vi "WPI_DigitalOutputDisablePWM.vi"(8 "error in (no error)":errorcluster, 11 "DigitalOutputDevRef":T1={"DIO Channel"=enum."DIO 1", "DevStatus"={"status"=FALSE, "code"=0, "source"=""}}) -> (0 "error out":errorcluster, 3 "DigitalOutputDevRef":T1={"DIO Channel"=enum."DIO 1", "DevStatus"={"status"=FALSE, "code"=0, "source"=""}})   [LabVIEW 2017]
doc: "Disable the generation of a PWM signal on a Digital Output channel.\n\nThis will stop generating a PWM signal and free 1 of the 6 PWM generators.\n\nThis software is licensed. Open the labview\\readme\\WPI Robotics Library Open Source License.txt file for more information."
uses:
  <vilib>/Rock Robotics/WPI/DigitalOutput/WPI_DigitalOutputDevRef.ctl
  <vilib>/Rock Robotics/SystemInterfaces/DIO/FPGA_DIOChannel.ctl
  <vilib>/Rock Robotics/WPI/DigitalModule/WPI_DigitalModuleDIOCacheOp.ctl
  <vilib>/Rock Robotics/SystemInterfaces/System/FPGA_SystemGet.vi
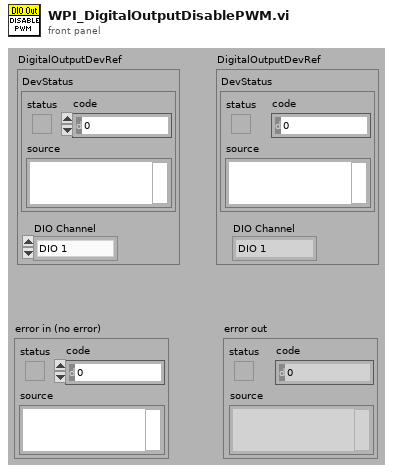
[diagram p1: front panel]
types:
  T1 = typedef "WPI_DigitalOutputDevRef.ctl" = cluster{"DIO Channel":T2, "DevStatus":errorcluster}
  T2 = typedef "FPGA_DIOChannel.ctl" = enum8{"DIO 0", "DIO 1", "DIO 2", "DIO 3", "DIO 4", "DIO 5", "DIO 6", "DIO 7", "DIO 8", "DIO 9", "DIO MXP 0", "DIO MXP 1", "DIO MXP 2", "DIO MXP 3", "DIO MXP 4", "DIO MXP 5", "DIO MXP 6", "DIO MXP 7", "DIO MXP 8", "DIO MXP 9", "DIO MXP 10", "DIO MXP 11", "DIO MXP 12", "DIO MXP 13", "DIO MXP 14", "DIO MXP 15", "SPI Port CS1", "SPI Port CS2", "SPI Port CS3", "SPI Port MISO", "SPI Port MOSI", "Invalid"}
  T3 = typedef "WPI_DigitalModuleDIOCacheOp.ctl" = enum16{"Acquire", "Release", "Status"}
  T4 = typedef "WPI_DigitalOutputPWMRef.ctl" = enum16{"DO PWM 0", "DO PWM 1", "DO PWM 2", "DO PWM 3", "DO PWM 4", "DO PWM 5", "Invalid"}
  T5 = typedef "FPGA_DIODevRef.ctl" = cluster{"DevStatus":errorcluster}
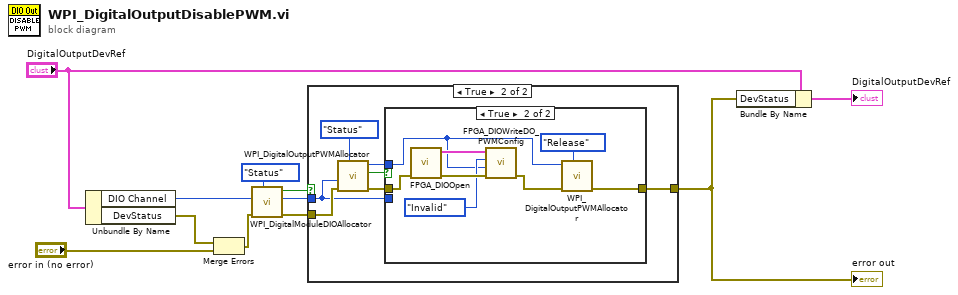
[diagram p0: block diagram]
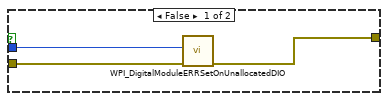
[diagram p2: hidden frame]
diagram:
  n1 = Unbundle By Name("DigitalOutputDevRef") -> ("DIO Channel"=w6:T2, "DevStatus"=w2:errorcluster)
  n2 = Merge Errors(w2, "error in (no error)") -> (w1:errorcluster)
  n3 = call <vilib>:"WPI_DigitalModuleDIOAllocator.vi"("AllocatedDIOMutex"=WPI_DigitalModuleDIOCacheOp."Status", "error in (no error)"=w1, "DIOChannel"=w6) -> ("error out"=w3:errorcluster, "Allocated DIOChannel"=w5:T2, "AllocatedDIO"=w4:bool)  [unwired: 1 in, 5 out]
  n4 = case shown="True" w4 {
    tunnel: [w13 w15] -> w8
    tunnel: w5 -> [w12 w17]
    tunnel: w3 -> [w14 w20]
    frame False {
      n5 = call <vilib>:"WPI_DigitalModuleERRSetOnUnallocatedDIO.vi"("error in (no error)"=w14, "DIOChannel"=w12) -> ("error out"=w13:errorcluster)  [unwired: 9 in]
    }
    frame True {
      n6 = call <vilib>:"WPI_DigitalOutputPWMAllocator.vi"("Operation"=WPI_DigitalModuleDIOCacheOp."Status", "error in (no error)"=w20, "DIO Channel"=w17) -> ("error out"=w18:errorcluster, "Allocated"=w19:bool, "PWM Allocated"=w16:T4)  [unwired: 2 in, 4 out]
      n7 = case shown="True" w19 {
        tunnel: w16 -> [_ w23]
        tunnel: w17 -> [_ _]
        tunnel: w18 -> [w22 w29]
        tunnel: [w22 w25] -> w15
        frame False {
        }
        frame True {
          n8 = call <vilib>:"FPGA_DIOOpen.vi"("error in (no error)"=w29) -> ("error out"=w28:errorcluster, "DIODeviceRef"=w30:T5)  [unwired: 1 in, 8 out]
          n9 = call <vilib>:"FPGA_DIOWriteDO_PWMConfig.vi"("error in (no error)"=w28, "DO_PWM Index"=w23, "DO_PWMOutputSelect"=FPGA_DIOChannel."Invalid", "DIODeviceRef"=w30) -> ("error out"=w24:errorcluster)  [unwired: 1 in, 6 out]
          n10 = call <vilib>:"WPI_DigitalOutputPWMAllocator.vi"("Operation"=WPI_DigitalModuleDIOCacheOp."Release", "error in (no error)"=w24, "PWM To Release"=w23) -> ("error out"=w25:errorcluster)  [unwired: 2 in, 6 out]
        }
      }
    }
  }
  "error out" <- w8
  n11 = Bundle By Name(cluster="DigitalOutputDevRef", "DevStatus"=w8) -> (→"DigitalOutputDevRef":T1)
